vi "test stage.vi"() -> ()   [LabVIEW 2010]
panel:
  in  "stop 2":bool
  in  "stop":bool
  out "Waveform Chart":cluster{"X out":dbl, "Y out":dbl, "Z out":dbl}(graph)
  out "out of range":bool
  in  "subsequent y move":dbl
  in  "initial x move":dbl format="%#_6p"
  in  "timeout":u32=100
  in  "Baud rate":u32=115200
  in  "VISA resource name":refnum<visa-resource-name>
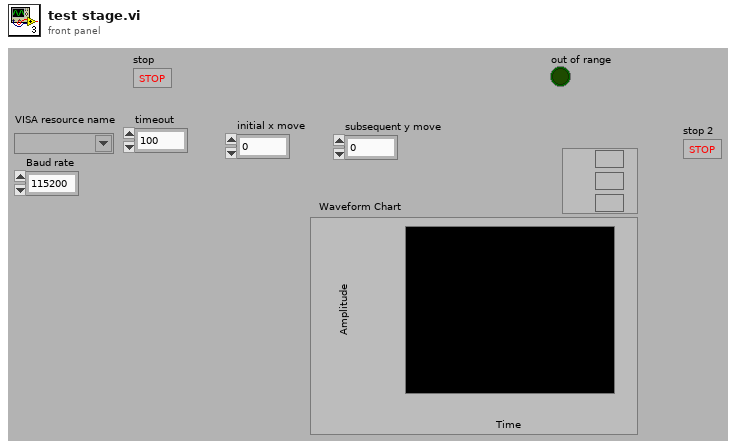
[diagram p1: front panel]
types:
  T1 = typedef "stage properties.ctl" = cluster{"VISA resource name":refnum<visa-resource-name>, "limits":cluster{"x max":dbl, "x min":dbl, "y max":dbl, "y min":dbl, "z max":dbl, "z min":dbl, "max vel (mm/s)":dbl}, "initialized":bool}
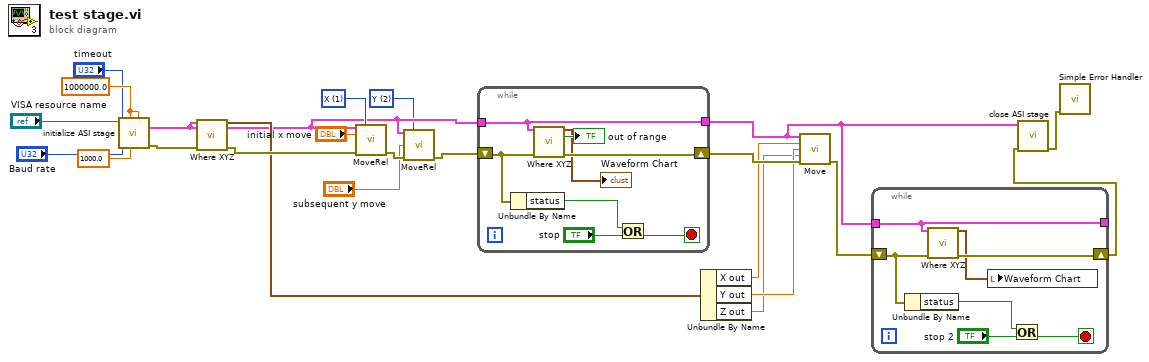
[diagram p0: block diagram]
diagram:
  w3 = u16 2 items=["No axis", "X", "Y", "Z", "XY", "XYZ"] ("Axis configuration")
  w17 = u16 1 items=["No axis", "X", "Y", "Z", "XY", "XYZ"] ("Axis configuration")
  w22 = 1000000.0 ("x range")
  n1 = call "initialize ASI stage.vi"("y range"=w22, "z range"=1000.0, "x range"=w22, "timeout"="timeout", "Baud rate"="Baud rate", "VISA resource name"="VISA resource name") -> ("error out"=w16:errorcluster, "ASI stage"=w4:T1)  [unwired: 4 in]
  n2 = call "Where XYZ.vi"("ASI stage"=w4, "error in (no error)"=w16) -> ("location"=w13:cluster{"X out":dbl, "Y out":dbl, "Z out":dbl}, "error out"=w15:errorcluster)  [unwired: 11 in, 1 out]
  n3 = call "MoveRel.vi"("ASI stage"=w4, "Axis configuration"=w17, "x"="initial x move", "error in (no error)"=w15) -> ("error out"=w5:errorcluster)  [unwired: 10 in, 1 out]
  n4 = call "MoveRel.vi"("ASI stage"=w4, "Axis configuration"=w3, "y"="subsequent y move", "error in (no error)"=w5) -> ("error out"=w1:errorcluster)  [unwired: 10 in, 1 out]
  n5 = while {
    shift-right: [w30] -> w14
    shift-left: w1 -> [w26]
    tunnel: w4 -> [w27]
    tunnel: [w27] -> w8
    stop <- w25 stop-if-true
    n6 = Unbundle By Name(w26) -> ("status"=w24:bool)
    n7 = call "Where XYZ.vi"("ASI stage"=w27, "error in (no error)"=w26) -> ("location"=→"Waveform Chart":cluster{"X out":dbl, "Y out":dbl, "Z out":dbl}, "out of range"=→"out of range":bool, "error out"=w30:errorcluster)  [unwired: 11 in]
    n8 = Or(x=w24, y="stop") -> (x .or. y?=w25:bool)
  }
  n9 = Unbundle By Name(w13) -> ("X out"=w12:dbl, "Y out"=w11:dbl, "Z out"=w10:dbl)
  n10 = call "Move.vi"("ASI stage"=w8, "x"=w12, "y"=w11, "z"=w10, "error in (no error)"=w14) -> ("error out"=w7:errorcluster)  [unwired: 9 in, 1 out]
  n11 = while {
    shift-right: [w38] -> w6
    shift-left: w7 -> [w35]
    tunnel: w8 -> [w36]
    tunnel: [w36] -> _
    stop <- w34 stop-if-true
    n12 = Unbundle By Name(w35) -> ("status"=w33:bool)
    n13 = call "Where XYZ.vi"("ASI stage"=w36, "error in (no error)"=w35) -> ("location"=w32:cluster{"X out":dbl, "Y out":dbl, "Z out":dbl}, "error out"=w38:errorcluster)  [unwired: 11 in, 1 out]
    n14 = local write "Waveform Chart"(w32) -> ()
    n15 = Or(x=w33, y="stop 2") -> (x .or. y?=w34:bool)
  }
  n16 = call "close ASI stage.vi"("error in (no error)"=w6, "ASI stage"=w8) -> ("error out"=w9:errorcluster)  [unwired: 8 in, 1 out]
  n17 = call <vilib>:"Simple Error Handler.vi"("error in (no error)"=w9) -> ()  [unwired: 4 in, 5 out]
